vi "Hide_Show Controls.vi"(10 "Hide?":bool, 11 "Controls":refnum<vi>[](array[refnum])) -> ()   [LabVIEW 2017, in "Engine Simulation Toolkit System Explorer.lvlib"]
uses:
  Engine Simulation Toolkit System Explorer.lvlib
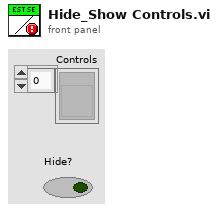
[diagram p1: front panel]
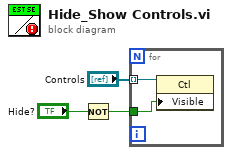
[diagram p0: block diagram]
diagram:
  n1 = Not(x="Hide?") -> (.not. x?=w1:bool)
  n2 = for {
    tunnel: "Controls" -> [w5] mode=indexing
    tunnel: w1 -> [w4]
    n3 = property class="Ctl"(reference=w5, "Visible"=w4) -> ()  [unwired: 1 in, 2 out]
  }
